vi "CAN Start Engine_STP_Engine.vi"(9 "ECU CAN Port":string="CAN2", 11 "Sequence Context":T1) -> (0 "error out":errorcluster)   [LabVIEW 2023, in "LTT_TeststandSteptypes.lvlib"]
uses:
  LTT_TeststandSteptypes.lvlib
  <vilib>/addons/TestStand/_TSLegacy.llb/LabVIEW Test - Sequence Context.ctl
  HardwareAbstractionLayer_LVOOP/Teststand/Teststand.lvclass
  HardwareAbstractionLayer_LVOOP/CAN/CAN Application Protocols/STP Protocol_class/STP Protocol.lvclass
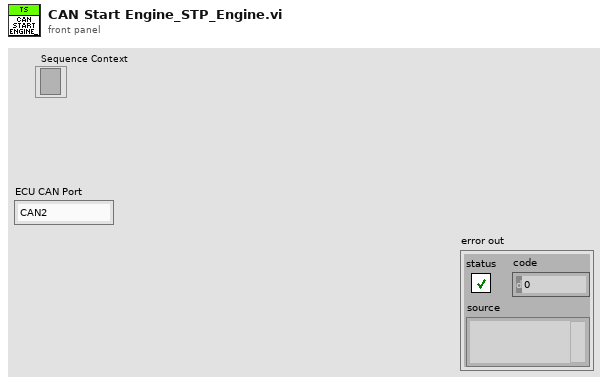
[diagram p1: front panel]
types:
  T1 = typedef "LabVIEW Test - Sequence Context.ctl" = refnum<k7>
  T2 = typedef "HardwareAbstractionLayer_LVOOP.lvlib/Teststand.lvclass/Teststand Status Control.ctl" = cluster{"Terminating or Aborting":bool, "Stop":bool, "Socket Count":i16, "Selected Sockets":i16[]}
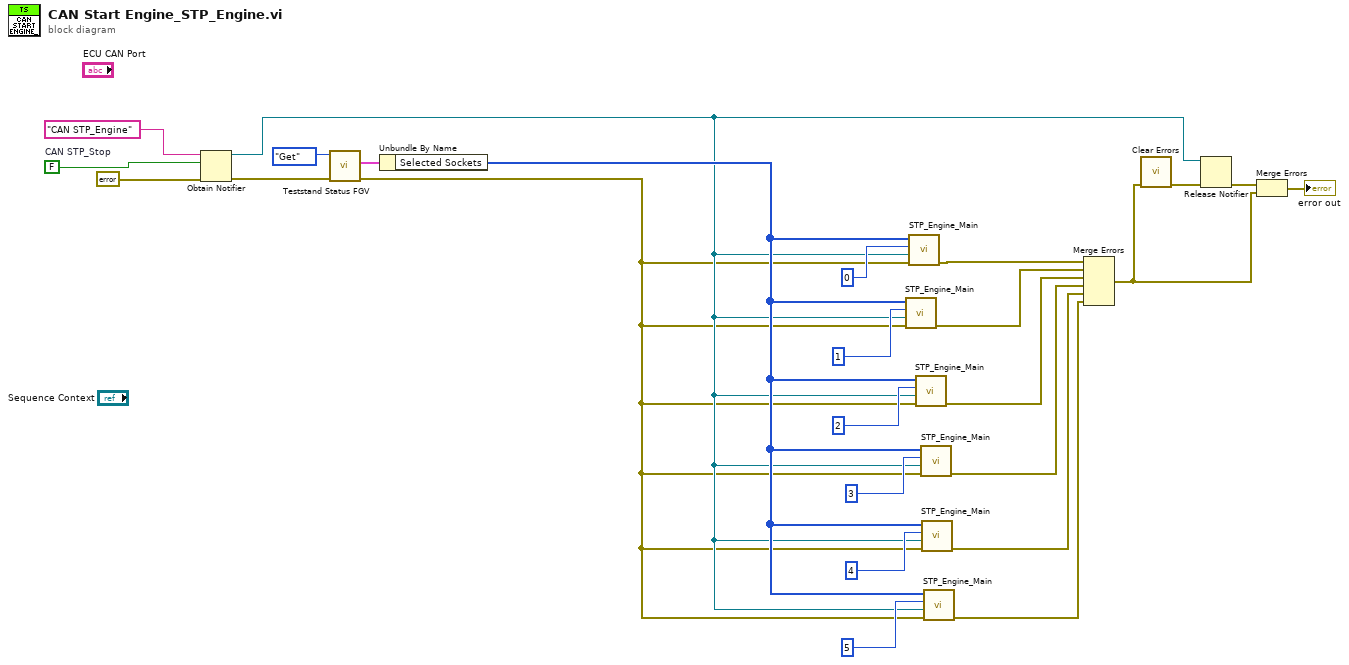
[diagram p0: block diagram]
diagram:
  w22 = FALSE  # CAN STP_Stop
  n1 = Obtain Notifier(name (unnamed)="CAN STP_Engine", notification data type=w22, error in (no error)=errorcluster {"status"=FALSE, "code"=0, "source"=""}) -> (notifier out=w6:refnum<notifier>, error out=w14:errorcluster)  [unwired: 1 in, 1 out]
  n2 = call "Teststand Status FGV.vi"("error in"=w14, "Option"=enum16{"Set", "Get"}."Get") -> ("error out"=w5:errorcluster, "Teststand Status Out"=w25:T2)  [unwired: 8 in]
  n3 = Unbundle By Name(w25) -> ("Selected Sockets"=w11:i16[])
  n4 = call "STP_Engine_Main.vi"("error in"=w5, "notifier in"=w6, "Socket No"=i16 1 ("Current Scoket"), "Selected Sockets"=w11) -> ("error out"=w12:errorcluster)  [unwired: 7 in]
  n5 = call "STP_Engine_Main.vi"("error in"=w5, "notifier in"=w6, "Socket No"=i16 0 ("Current Scoket"), "Selected Sockets"=w11) -> ("error out"=w15:errorcluster)  [unwired: 7 in]
  n6 = call "STP_Engine_Main.vi"("error in"=w5, "notifier in"=w6, "Socket No"=i16 2 ("Current Scoket"), "Selected Sockets"=w11) -> ("error out"=w4:errorcluster)  [unwired: 7 in]
  n7 = call "STP_Engine_Main.vi"("error in"=w5, "notifier in"=w6, "Socket No"=i16 3 ("Current Scoket"), "Selected Sockets"=w11) -> ("error out"=w3:errorcluster)  [unwired: 7 in]
  n8 = call "STP_Engine_Main.vi"("error in"=w5, "notifier in"=w6, "Socket No"=i16 4 ("Current Scoket"), "Selected Sockets"=w11) -> ("error out"=w2:errorcluster)  [unwired: 7 in]
  n9 = call "STP_Engine_Main.vi"("error in"=w5, "notifier in"=w6, "Socket No"=i16 5 ("Current Scoket"), "Selected Sockets"=w11) -> ("error out"=w1:errorcluster)  [unwired: 7 in]
  n10 = Merge Errors(w15, w12, w4, w3, w2, w1) -> (w17:errorcluster)
  n11 = call <vilib>:"Clear Errors.vi"("error in (no error)"=w17) -> ("error out"=w19:errorcluster)  [unwired: 5 in, 1 out]
  n12 = Release Notifier(notifier=w6, error in (no error)=w19) -> (error out=w18:errorcluster)  [unwired: 1 in, 2 out]
  n13 = Merge Errors(w18, w17) -> (→"error out":errorcluster)
